vi "Read output channels.vi"(8 "error in (no error)":errorcluster, 11 "Scaling runtime in":refnum<class "Scaling runtime.lvclass">) -> (0 "error out":errorcluster, 2 "output channels":cluster{"data type":T1, "index":i32}[][](array[cluster]), 3 "Scaling runtime out":refnum<class "Scaling runtime.lvclass">)   [LabVIEW 2013, in "Scaling runtime.lvclass"]
uses:
  Scaling runtime.lvclass
  <vilib>/NI/Tag Bus/tag/Data Type.ctl
  <vilib>/NI/Tag Bus/tag/tag descriptor.lvclass
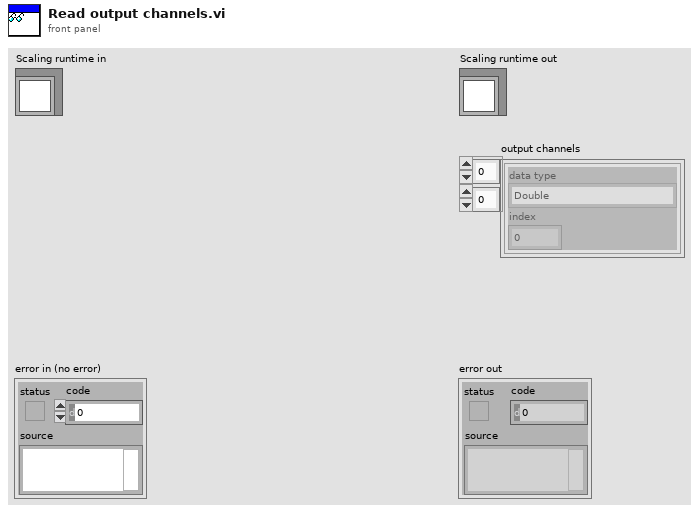
[diagram p1: front panel]
types:
  T1 = typedef "tag bus.lvlib/tag descriptor.lvclass/Data Type.ctl" = enum16{"Double", "Single", "I64", "I32", "I16", "I8", "U64", "U32", "U16", "U8", "Boolean", "String", "Array of Double", "Array of Single", "Array of I64", "Array of I32", "Array of I16", "Array of I8", "Array of U64", "Array of U32", "Array of U16", "Array of U8", "Array of Boolean", "Array of String"}
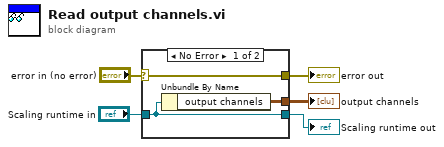
[diagram p0: block diagram]
diagram:
  n1 = case shown="No Error" "error in (no error)" {
    selector: "error in (no error)" -> [w8 w9]
    tunnel: [w8 w9] -> w4
    tunnel: [w7 w10] -> w2
    tunnel: "Scaling runtime in" -> [w7 w10]
    tunnel: [w6 _] -> w1
    frame No Error {
      n2 = Unbundle By Name(w7) -> ("output channels"=w6:cluster{"data type":T1, "index":i32}[][])
    }
    frame Error {
    }
  }
  "error out" <- w4
  "Scaling runtime out" <- w2
  "output channels" <- w1
